vi "solar_voy Obtain.vi"(6 "Suppress Errors? (T)":bool=TRUE, 8 "error in (no error)":errorcluster, 9 "Create if not found? (T)":bool=TRUE, 11 "Interface Name":string) -> (0 "error out":errorcluster, 1 "Created New?":bool, 3 "Voyager Refnum":T1)   [LabVIEW 2018]
doc: "This obtains a Voyager reference by name. The Voyager reference names prefix 'solar_voyager_' to ensure unique namespaces."
uses:
  solar_voy_ctl Voyager.ctl
  type/solar_type Item Type.ctl
  solar_voy_def/solar_voy_def_ctl ITEM TYPE.ctl
  solar_voy_def/solar_voy_def_ctl ITEM.ctl
  solar_voy_def/solar_voy_def_ctl PACKET.ctl
  solar_voy_def/solar_voy_def_ctl PACKET_ID.ctl
  solar_voy_def/solar_voy_def_ctl HDR.ctl
  solar_voy_ctl TCP.ctl
  solar_voy_ctl Port Setup.ctl
  solar_voy_ctl Voyager Refnum.ctl
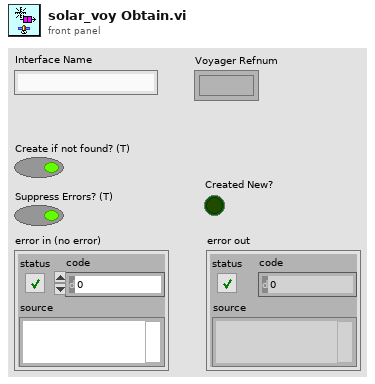
[diagram p1: front panel]
types:
  T1 = typedef "solar_voy_ctl Voyager Refnum.ctl" = refnum<k1>
  T2 = typedef "solar_voy_ctl Voyager.ctl" = cluster{"PACKETS":T3[], "COSMOS_Root":path, "CMD_HDR":T8, "TLM_HDR":T8, "TCPs":T9[], "VoyagerIDOffset":cluster{"VoyagerIDOffset":u16[], "Target Names":string[]}}
  T3 = typedef "solar_voy_def_ctl PACKET.ctl" = cluster{"PACKET_ID":T4, "ENDIAN":enum8{"BIG", "LITTLE"}, "DESC":string, "HZRD":bool, "ITEMS":T5[], "NoExport":bool, "last_time":timestamp, "last_count":u32, "last_data":string}
  T4 = typedef "solar_voy_def_ctl PACKET_ID.ctl" = cluster{"ID":u16, "CMD":enum8{"CMD", "TLM"}, "TARGET":string, "PACKET":string}
  T5 = typedef "solar_voy_def_ctl ITEM.ctl" = cluster{"NAME":string, "OFFSET":i32, "SIZE":i32, "TYPE":T6, "EACH_SIZE":i32, "LVTYPE":T7, "MIN":dbl, "MAX":dbl, "DEFAULT":string, "DESC":string, "ID":bool, "MODIFIERS":variant, "last_value":variant}
  T6 = typedef "solar_voy_def_ctl ITEM TYPE.ctl" = enum8{"BLOCK", "INT", "UINT", "FLOAT", "STRING"}
  T7 = typedef "solar_type Item Type.ctl" = enum16{"NULL", "UNKNOWN", "CLUSTER", "I8", "I16", "I32", "I64", "U8", "U16", "U32", "U64", "U8_ENUM", "U16_ENUM", "U32_ENUM", "SGL", "DBL", "BOOLEAN", "STRING", "PATH", "VISA", "TAG", "TIME", "I8_1D", "I16_1D", "I32_1D", "I64_1D", "U8_1D", "U16_1D", "U32_1D", "U64_1D", "U8_ENUM_1D", "U16_ENUM_1D", "U32_ENUM_1D", "SGL_1D", "DBL_1D", "BOOLEAN_1D", "STRING_1D", "PATH_1D", "VISA_1D", "TAG_1D", "TIME_1D", "I8_2D", "I16_2D", "I32_2D", "I64_2D", "U8_2D", "U16_2D", "U32_2D", "U64_2D", "U8_ENUM_2D", "U16_ENUM_2D", "U32_ENUM_2D", "SGL_2D", "DBL_2D", "BOOLEAN_2D", "STRING_2D", "PATH_2D", "VISA_2D", "TAG_2D", "TIME_2D"}
  T8 = typedef "solar_voy_def_ctl HDR.ctl" = cluster{"ITEMS":T5[], "LENGTH_NAME":string, "LENGTH_VALUE_OFFSET":i32, "ID_NAME":string, "ENDIAN":enum8{"BIG", "LITTLE"}, "GUID_NAME":string, "DEFAULT_TARGET":string, "DEFAULT_PACKET":string, "DEFAULT_ERROR":string}
  T9 = typedef "solar_voy_ctl TCP.ctl" = cluster{"Connected":bool, "Port":u16, "Listener":refnum<k5>, "ServerIP":string, "TCP":refnum<k5>, "Setup":T10, "VIRefnum":refnum<vi>, "TARGETS_CMD":string[], "TARGETS_TLM":string[]}
  T10 = typedef "solar_voy_ctl Port Setup.ctl" = enum8{"SERVER", "CLIENT", "SERVER_CMD", "SERVER_TLM"}
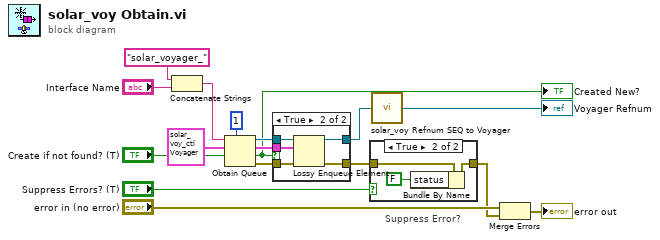
[diagram p0: block diagram]
diagram:
  w11 = T2 {"PACKETS"=[], "COSMOS_Root"=path "", "CMD_HDR"={"ITEMS"=[], "LENGTH_NAME"="", "LENGTH_VALUE_OFFSET"=0, "ID_NAME"="", "ENDIAN"=enum."BIG", "GUID_NAME"="", "DEFAULT_TARGET"="", "DEFAULT_PACKET"="", "DEFAULT_ERROR"=""}, "TLM_HDR"={"ITEMS"=[], "LENGTH_NAME"="", "LENGTH_VALUE_OFFSET"=0, "ID_NAME"="", "ENDIAN"=enum."BIG", "GUID_NAME"="", "DEFAULT_TARGET"="", "DEFAULT_PACKET"="", "DEFAULT_ERROR"=""}, "TCPs"=[], "VoyagerIDOffset"={"VoyagerIDOffset"=[], "Target Names"=[]}} ("TCP Voyager")
  n1 = Concatenate Strings("solar_voyager_", "Interface Name") -> (w14:string)
  n2 = Obtain Queue(max queue size (-1, unlimited)=1, name (unnamed)=w14, element data type=w11, create if not found? (T)="Create if not found? (T)") -> (queue out=w12:refnum<queue>, created new?=w2:bool, error out=w10:errorcluster)  [unwired: 1 in]
  "Created New?" <- w2
  n3 = case shown="True" w2 {
    tunnel: w12 -> [w18 w23]
    tunnel: w11 -> [_ w19]
    tunnel: w10 -> [w17 w22]
    tunnel: [w18 w21] -> w9
    tunnel: [w17 w20] -> w8
    frame False {
    }
    frame True {
      n4 = Lossy Enqueue Element(queue=w23, element=w19, error in (no error)=w22) -> (queue out=w21:refnum<queue>, error out=w20:errorcluster)  [unwired: 2 out]
    }
  }
  n5 = case "Suppress Error?" shown="True" "Suppress Errors? (T)" {
    tunnel: w8 -> [w24 w27]
    tunnel: [w24 w26] -> w5
    frame False {
    }
    frame True {
      n6 = Bundle By Name(cluster=w27, "status"=FALSE) -> (w26:errorcluster)
    }
  }
  n7 = call "solar_voy Refnum SEQ to Voyager.vi"("Voyager SEQ"=w9) -> ("Voyager Refnum"=→"Voyager Refnum":T1)
  n8 = Merge Errors("error in (no error)", w5) -> (→"error out":errorcluster)
